vi "DB Connection handler.vi"(8 "error in (no error)":errorcluster, 11 "DB Action":enum16{"Create", "Close", "Get"}(ring)=enum."Get") -> (0 "error out":errorcluster, 3 "connection reference":T1)   [LabVIEW 2018]
uses:
  <vilib>/addons/database/Connection.llb/Conn ObjectReference.ctl
  <vilib>/addons/database/Connection.llb/DB Tools Open Connec (String).vi
  <vilib>/addons/database/NI_Database_API.lvlib
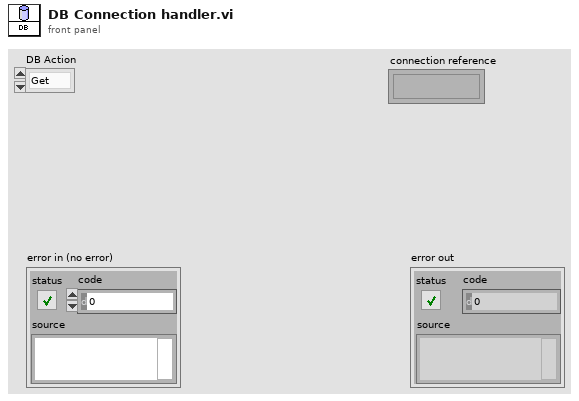
[diagram p1: front panel]
types:
  T1 = typedef "NI_Database_API.lvlib/Conn ObjectReference.ctl" = refnum<k1>
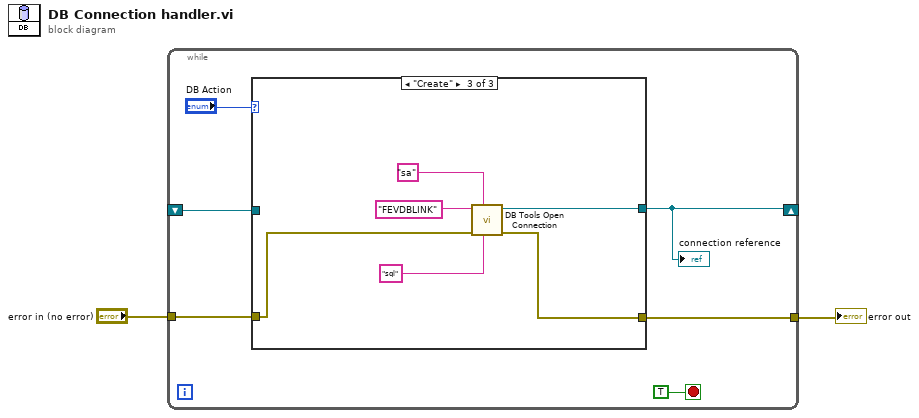
[diagram p0: block diagram]
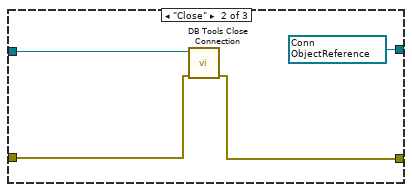
[diagram p3: hidden frame]
diagram:
  n1 = while {
    tunnel: [w7] -> w1
    tunnel: "error in (no error)" -> [w6]
    shift-right: [w3] -> _
    shift-left: _ -> [w4]
    stop <- TRUE stop-if-true
    n2 = case shown="\"Create\"" "DB Action" {
      tunnel: [w9 w12 w17] -> w7
      tunnel: w6 -> [w9 w13 w16]
      tunnel: [w10 w11 w15] -> w3
      tunnel: w4 -> [w10 w14 _]
      frame "Get", Default {
      }
      frame "Close" {
        w11 = T1 refnum items=["Connection"] ("connection reference")
        n3 = call <vilib>:"DB Tools Close Connection.vi"("error in (no error)"=w13, "connection reference"=w14) -> ("error out"=w12:errorcluster)  [unwired: 5 in]
      }
      frame "Create" {
        n4 = call-poly <vilib>:"DB Tools Open Connection.vi"("password"="sql", "userID"="sa", "error in (no error)"=w16, "connection information"="FEVDBLINK") -> ("error out"=w17:errorcluster, "connection reference"=w15:T1)  [unwired: 4 in]
      }
    }
    "connection reference" <- w3
  }
  "error out" <- w1
